vi "MAIN_init_autofocus.vi"(0 "Start acquisition":bool, 1 "queue piezo":refnum<queue>, 2 "queue FPGA":refnum<queue>, 5 "Measure QPD":bool caption="Calibration", 7 "PID gains":T2={"proportional gain (Kc)"=50.0, "integral time (Ti, min)"=0.03, "derivative time (Td, min)"=0.0} {"derivative time (Td, min)" format="%.3f"; "integral time (Ti, min)" format="%.3f"; "proportional gain (Kc)" format="%.3f"}, 11 "error in":errorcluster, 12 "Switch":bool, 13 "Init":bool, 14 "Autotune?":bool) -> (4 "Next task":T1, 15 "error out":errorcluster)   [LabVIEW 2015]
uses:
  CONTROLS/Q_FPGA_element.ctl
  CONTROLS/Q_MCL_piezo_element.ctl
  CONTROLS/Q_main_element.ctl
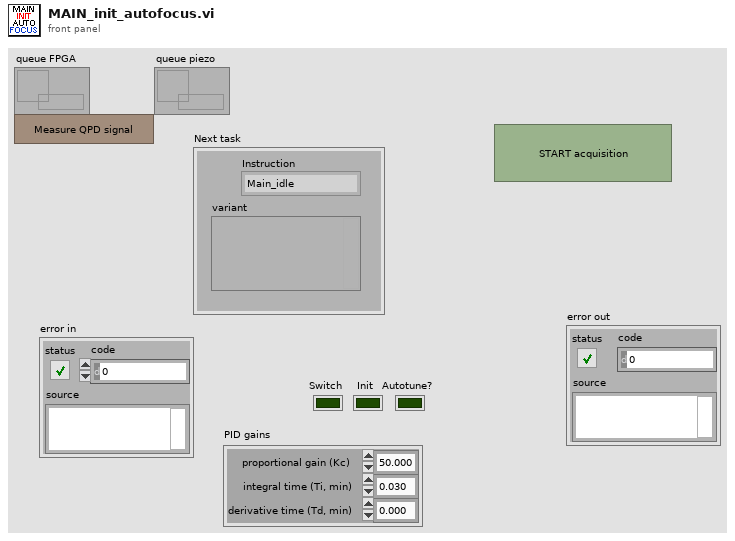
[diagram p1: front panel]
types:
  T1 = typedef "Q_main_element.ctl" = cluster{"variant":variant, "Instruction":enum16{"Main_idle", "Main_initialize", "Main_initialize_TDMS", "Main_initialize_Queue", "Main_error", "Main_DAQ_initialization_results", "Main_ASI_initialization_results", "Main_Piezo_initialization_results", "Main_Valve_initialization_results", "Main_Pump_initialization_results", "Main_CAMERA_initialization_results", "Main_FPGA_initialization_results", "Main_DAQ_error", "Main_ASI_error", "Main_Piezo_error", "Main_CAMERA_error", "Main_Valve_error", "Main_Pump_error", "Main_FPGA_error", "Main_start_acquiring", "Main_not_acquiring", "Main_acquiring", "Main_stop_acquiring", "Main_change_exposure", "Main_change_z_scan_parameters", "Main_define_ROI", "Main_define_mosaic", "Main_read_kinetic_time", "Main_cooler", "Main_read_temperature", "Main_save_XY", "Main_load_XY", "Main_discard_XY", "Main_move_to_XY", "Main_measure_QPD", "Main_autofocus_calibration", "Main_autofocus_initialization", "Main_autofocus_stop", "Main_save_PID", "Main_change_H_valve_position", "Main_two_way_valve", "Main_save_movie", "Main_init_single_scan", "Main_single_scan", "Main_stop_single_scan", "Main_merFISH_illumination_parameters", "Main_merFISH_buffer_probe_list", "Main_merFISH_injections_procedure", "Main_merFISH_save_setpoint", "Main_merFISH_DAPI_parameters", "Main_merFISH_Brightfield_parameters", "Main_merFISH_save_embryo_ROI", "Main_merFISH_init", "Main_merFISH_resume", "Main_merFISH_start_autofocus", "Main_merFISH_open_close_valve_merFISH", "Main_merFISH_open_close_valve_photobleaching", "Main_merFISH_hybridization", "Main_merFISH_move_to_ROI", "Main_merFISH_wait_stabilization", "Main_merFISH_move_to_REF", "Main_merFISH_scan", "Main_merFISH_photobleaching_injection", "Main_merFISH_photobleaching", "Main_merFISH_send_email", "Main_merFISH_close", "Main_STOP"}}
  T2 = cluster{"proportional gain (Kc)":dbl, "integral time (Ti, min)":dbl, "derivative time (Td, min)":dbl}
  T3 = typedef "Q_FPGA_element.ctl" = cluster{"variant":variant, "Instruction":enum16{"FPGA_idle", "FPGA_initialize", "FPGA_error", "FPGA_security_stop", "FPGA_laser", "FPGA_start_stop_measure_QPD", "FPGA_measure_QPD", "FPGA_measure_QPD_noise", "FPGA_stop_measure_QPD", "FPGA_init_autofocus", "FPGA_init_single_scan", "FPGA_stop_single_scan", "FPGA_init_merFISH", "FPGA_measure_QPD_merFISH", "FPGA_init_scan_merFISH", "FPGA_scan_merFISH", "FPGA_close_merFISH", "FPGA_stop"}}
  T4 = typedef "Q_MCL_piezo_element.ctl" = cluster{"variant":variant, "Instruction":enum16{"Piezo_idle", "Piezo_initialize", "Piezo_error", "Piezo_security_stop", "Piezo_read_z", "Piezo_move_z", "Piezo_keyboard_move", "Piezo_close_autofocus_calibration_ramp", "Piezo_change_init_state", "Piezo_init_autofocus", "Piezo_init_autofocus_merFISH_TL", "Piezo_autofocus", "Piezo_autofocus_merFISH_TL", "Piezo_stop_autofocus", "Piezo_stop_autofocus_merFISH_TL", "Piezo_autofocus_lost", "Piezo_resume_autofocus_merFISH_TL", "Piezo_check_z_position_merFISH_TL", "Piezo_init_ramp", "Piezo_move_z_ramp", "Piezo_close_ramp", "Piezo_close_merFISH", "Piezo_stop"}}
  T5 = cluster{"Init":bool, "Switch":bool, "Autotune?":bool, "PID gains":cluster{"proportional gain (Kc)":dbl, "integral time (Ti, min)":dbl, "derivative time (Td, min)":dbl}}
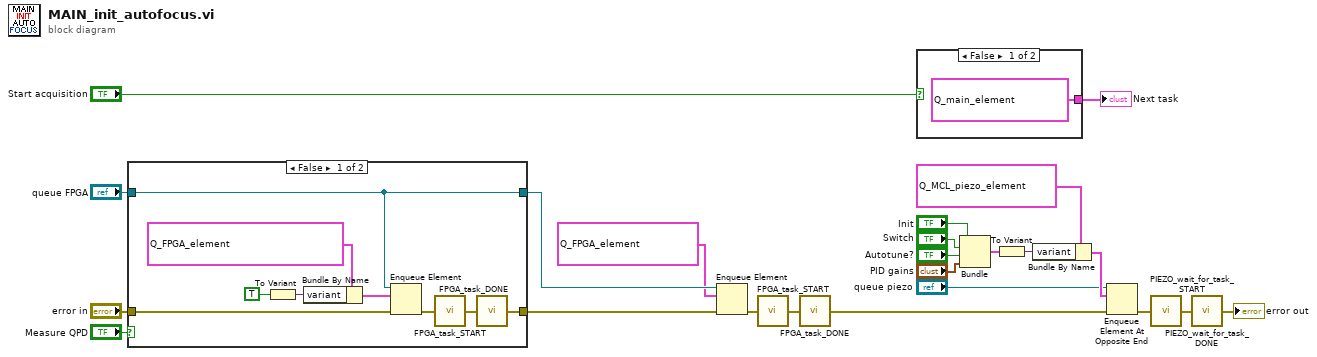
[diagram p0: block diagram]
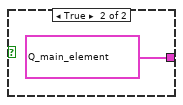
[diagram p2: hidden frame]
diagram:
  n1 = case shown="False" "Measure QPD" {
    tunnel: "error in" -> [w32 w34]
    tunnel: "queue FPGA" -> [w24 w33]
    tunnel: [w25 w34] -> w6
    tunnel: [w24 w33] -> w5
    frame False {
      n2 = To Variant(anything=TRUE) -> (Variant=w29:variant)
      n3 = Bundle By Name(cluster=T3 {"variant"=variant, "Instruction"=enum."FPGA_start_stop_measure_QPD"} ("element"), "variant"=w29) -> (w28:T3)
      n4 = Enqueue Element(queue=w24, element=w28, error in (no error)=w32) -> (error out=w27:errorcluster)  [unwired: 1 in, 2 out]
      n5 = call "FPGA_task_START.vi"("error in"=w27) -> ("error out"=w26:errorcluster)
      n6 = call "FPGA_task_DONE.vi"("error in"=w26) -> ("error out"=w25:errorcluster)
    }
    frame True {
    }
  }
  n7 = Enqueue Element(queue=w5, element=T3 {"variant"=variant, "Instruction"=enum."FPGA_init_autofocus"}, error in (no error)=w6) -> (error out=w3:errorcluster)  [unwired: 1 in, 2 out]
  n8 = call "FPGA_task_START.vi"("error in"=w3) -> ("error out"=w2:errorcluster)
  n9 = call "FPGA_task_DONE.vi"("error in"=w2) -> ("error out"=w1:errorcluster)
  n10 = case shown="False" "Start acquisition" {
    tunnel: [T1 {"variant"=variant, "Instruction"=enum."Main_not_acquiring"} ("Q_main_element") T1 {"variant"=variant, "Instruction"=enum."Main_acquiring"} ("Q_main_element")] -> w8
    frame False {
    }
    frame True {
    }
  }
  "Next task" <- w8
  n11 = Bundle("Init"="Init", "Switch"="Switch", "Autotune?"="Autotune?", "PID gains"="PID gains") -> (w18:T5)  [unwired: 1 in]
  n12 = To Variant(anything=w18) -> (Variant=w19:variant)
  n13 = Bundle By Name(cluster=T4 {"variant"=variant, "Instruction"=enum."Piezo_init_autofocus"} ("element"), "variant"=w19) -> (w20:T4)
  n14 = Enqueue Element At Opposite End(queue="queue piezo", element=w20, error in (no error)=w1) -> (error out=w22:errorcluster)  [unwired: 1 in, 2 out]
  n15 = call "PIEZO_wait_for_task_START.vi"("error in"=w22) -> ("error out"=w23:errorcluster)
  n16 = call "PIEZO_wait_for_task_DONE.vi"("error in"=w23) -> ("error out"=→"error out":errorcluster)
